vi "Create Log File.vi"(8 "error in (no error)":errorcluster, 10 "Info":T1, 11 "Current Folder":path) -> (0 "error out":errorcluster, 3 "Log File Name":path)   [LabVIEW 2014]
uses:
  Controls/Info.ctl
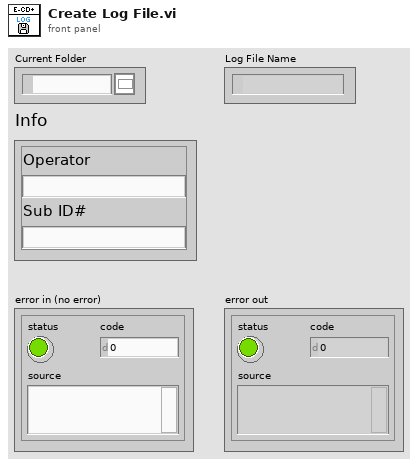
[diagram p1: front panel]
types:
  T1 = typedef "Info.ctl" = cluster{"Operator":string, "Sub ID#":string}
  T2 = enum16{"open", "replace", "create", "open or create", "replace or create", "replace or create with confirmation"}
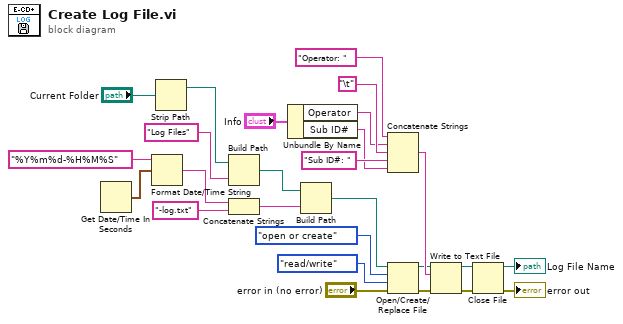
[diagram p0: block diagram]
diagram:
  n1 = Get Date/Time In Seconds() -> (seconds since 1Jan1904=w7:timestamp)
  n2 = Format Date/Time String(time format string (%c)="%Y%m%d-%H%M%S", seconds (now)=w7) -> (date/time string=w10:string)  [unwired: 1 out]
  n3 = Strip Path(path="Current Folder") -> (stripped path=w5:path)  [unwired: 1 out]
  n4 = Build Path(base path=w5, name or relative path="Log Files") -> (appended path=w9:path)
  n5 = Concatenate Strings(w10, "-log.txt" ("string")) -> (w12:string)
  n6 = Unbundle By Name("Info") -> ("Operator"=w2:string, "Sub ID#"=w1:string)
  n7 = Build Path(base path=w9, name or relative path=w12) -> (appended path=w25:path)
  n8 = Concatenate Strings("Operator: " ("string"), w2, "\t", "Sub ID#: " ("string"), w1) -> (w22:string)
  n9 = Open/Create/Replace File(file path (use dialog)=w25, error in="error in (no error)", operation (0:open)=T2."open or create", access (0:read/write)=enum16{"read/write", "read-only", "write-only"}."read/write") -> (refnum out=w16:refnum<file>, error out=w15:errorcluster)  [unwired: 2 in, 1 out]
  n10 = Write to Text File(file (use dialog)=w16, text=w22, error in=w15) -> (refnum out=w18:refnum<file>, error out=w17:errorcluster)  [unwired: 1 in, 1 out]
  n11 = Close File(refnum=w18, error in=w17) -> (path=→"Log File Name":path, error out=→"error out":errorcluster)
